vi "Get Glyph.vi"(8 "error in (no error)":errorcluster, 11 "glyph slot ref in":i64) -> (0 "error out":errorcluster, 2 "glyph ref out":i64, 3 "glyph slot ref":i64)   [LabVIEW 2023, in "Freetype Drawer.lvlib"]
uses:
  Freetype Drawer.lvlib
  libfreetype.dll
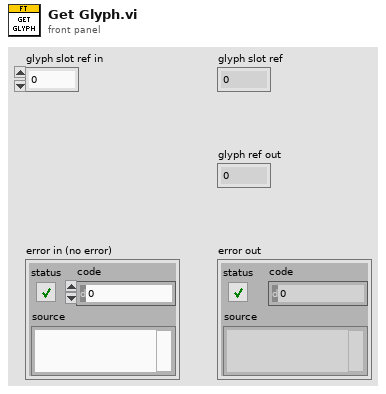
[diagram p1: front panel]
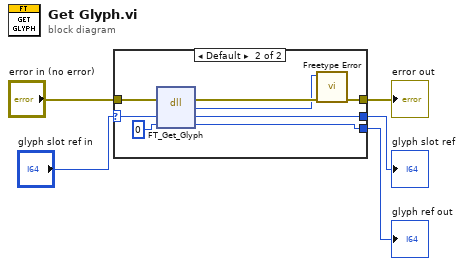
[diagram p0: block diagram]
diagram:
  n1 = case shown="Default" "glyph slot ref in" {
    selector: "glyph slot ref in" -> [w6 w13]
    tunnel: [_ w15] -> w5
    tunnel: "error in (no error)" -> [w7 w14]
    tunnel: [w6 w12] -> w2
    tunnel: [w7 w8] -> w1
    frame 0 {
    }
    frame Default {
      n2 = dll-call lib="E:/Labview/LV 2023/Libs/LV Symbol/Freetype Drawer/libfreetype.dll" fn="FT_Get_Glyph"(error in=w14, "glyph in"=w13, "glyph ref out"=i64 0) -> (error out=w10:errorcluster, "error"=w9:i32, "glyph in"=w12:i64, "glyph ref out"=w15:i64)  [unwired: 2 in, 1 out]
      n3 = call "Freetype Error.vi"("error in (no error)"=w10, "Error"=w9) -> ("error out"=w8:errorcluster)  [unwired: 9 in]
    }
  }
  "error out" <- w1
  "glyph ref out" <- w5
  "glyph slot ref" <- w2
